vi "Convert Version.vi"(8 "error in (no error)":errorcluster, 11 "Version":string) -> (0 "error out":errorcluster, 3 "Build Specification Version":T1)   [LabVIEW 2015, in "ExecuteAllBuildSpecsWithVersion.lvclass"]
uses:
  ExecuteAllBuildSpecsWithVersion.lvclass
  <vilib>/AppBuilder/AB_API_Simple/Build Specification Version.ctl
  <vilib>/AppBuilder/AB_API_Simple/NI_App_Builder_API.lvlib
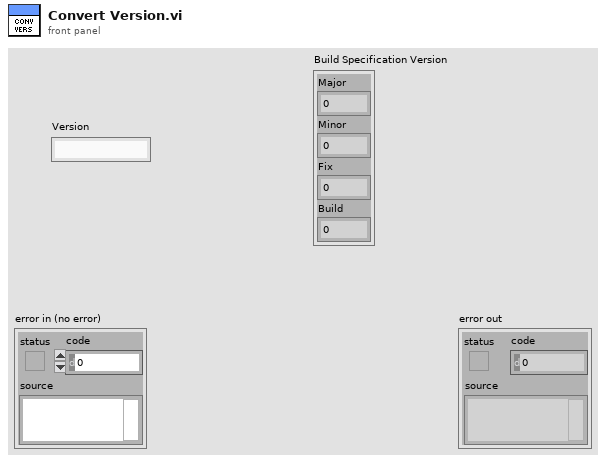
[diagram p1: front panel]
types:
  T1 = typedef "NI_App_Builder_API.lvlib/Build Specification Version.ctl" = cluster{"Major":u16, "Minor":u16, "Fix":u16, "Build":u16}
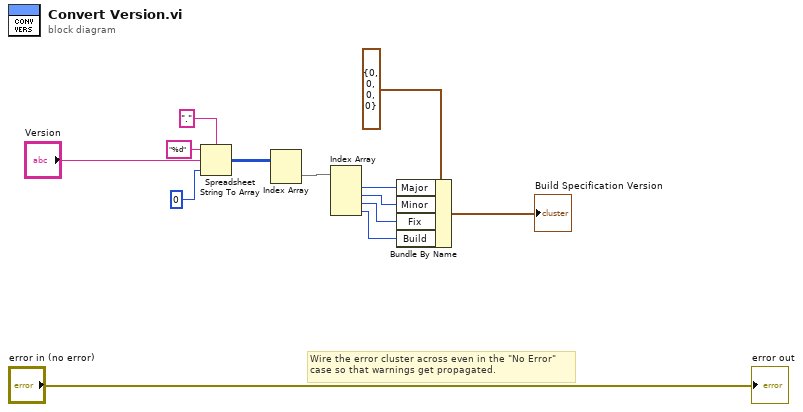
[diagram p0: block diagram]
diagram:
  # "Wire the error cluster across even in the \"No Error\"\ncase so that warnings get propagated."
  n1 = Spreadsheet String To Array(delimiter (Tab)=".", format string="%d", spreadsheet string="Version", array type (2D Dbl)=u16 0) -> (array=w9:u16[][])
  n2 = Index Array(array=w9) -> (element=w8:u16[])  [unwired: 2 in]
  n3 = Index Array(array=w8) -> (element #1=w6:u16, element #2=w3:u16, element #3=w2:u16, element #4=w1:u16)  [unwired: 4 in]
  n4 = Bundle By Name(cluster=T1 {"Major"=0, "Minor"=0, "Fix"=0, "Build"=0} ("Build Specification Version"), "Major"=w6, "Minor"=w3, "Fix"=w2, "Build"=w1) -> (→"Build Specification Version":T1)
  "error out" <- "error in (no error)"
